vi "svc_Mag2 to Mag Spectrum.vi"(4 "power spectrum":cluster{"f0":dbl, "df":dbl, "spectrum":dbl[]} {"spectrum" format="%.2f"; "df" format="%.2f"; "f0" format="%.2f"}) -> (1 "magnitude spectrum":cluster{"f0":dbl, "df":dbl, "spectrum":dbl[]} {"spectrum" format="%.2f"; "df" format="%.2f"; "f0" format="%.2f"})   [LabVIEW 2017]
panel:
  # "spectrum must have linear (not dB) scale"
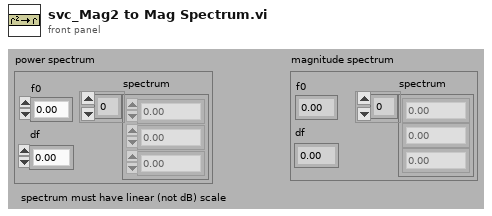
[diagram p1: front panel]
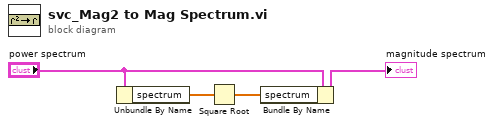
[diagram p0: block diagram]
diagram:
  n1 = Unbundle By Name("power spectrum") -> ("spectrum"=w2:dbl[])
  n2 = Square Root(x=w2) -> (sqrt(x)=w1:dbl[])
  n3 = Bundle By Name(cluster="power spectrum", "spectrum"=w1) -> (→"magnitude spectrum":cluster{"f0":dbl, "df":dbl, "spectrum":dbl[]})
